vi "Set Column as Default.vi"(8 "error in (no error)":errorcluster, 10 "Default Column (T)?":bool=TRUE, 11 "Composed Column in":refnum<class "Composed Column.lvclass">) -> (0 "error out":errorcluster, 3 "Composed Column out":refnum<class "Composed Column.lvclass">)   [LabVIEW 2020, in "Composed Columns.lvlib" / "Composed Column.lvclass"]
uses:
  Composed Column.lvclass
  Composed Column.lvclass/Composed Column.ctl
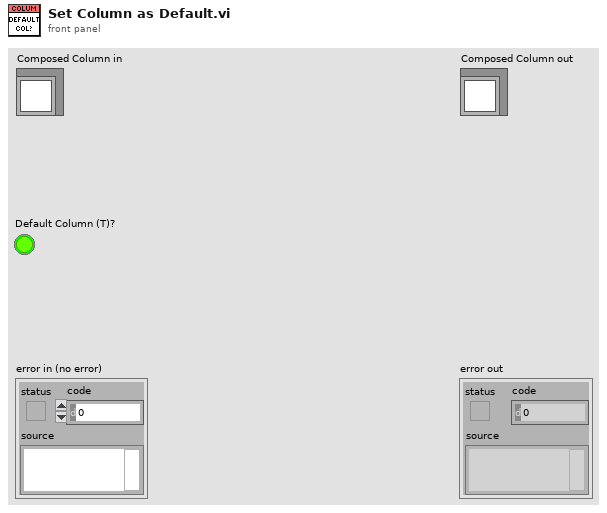
[diagram p1: front panel]
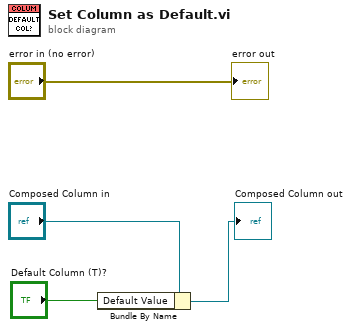
[diagram p0: block diagram]
diagram:
  n1 = Bundle By Name(cluster="Composed Column in", "Default Value"="Default Column (T)?") -> (→"Composed Column out":refnum<class "Composed Column.lvclass">)
  "error out" <- "error in (no error)"
